vi "translateDigitalInputs.vi"(0 "Controller in":refnum<class "_Controller.lvclass">, 2 "di_value (in)":u32, 5 "error in (no error)":errorcluster) -> (14 "Controller out":refnum<class "_Controller.lvclass">, 16 "dig_in_value (out)":u32, 17 "dig_in_items (out)":T1[](array[typedef]), 19 "error out":errorcluster)   [LabVIEW 2020, in "classes.lvlib" / "_Controller.lvclass"]
uses:
  _Controller.lvclass
  digital_input_item.ctl
  digital_input.ctl
  common.lvlib
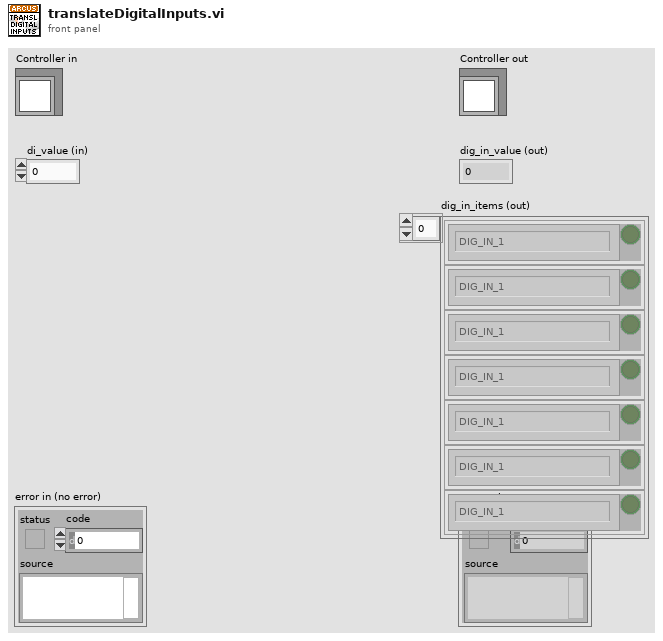
[diagram p1: front panel]
types:
  T1 = typedef "common.lvlib/digital_input_item.ctl" = cluster{"item":T2, "status":bool}
  T2 = typedef "common.lvlib/digital_input.ctl" = enum16{"DIG_IN_1", "DIG_IN_2", "DIG_IN_3", "DIG_IN_4", "DIG_IN_5", "DIG_IN_6", "DIG_IN_7", "DIG_IN_8", "NEG_LIMIT", "HOME", "POS_LIMIT"}
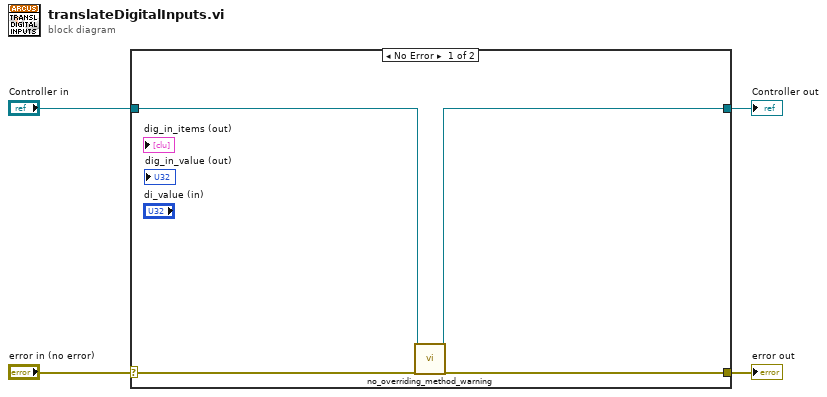
[diagram p0: block diagram]
diagram:
  n1 = case shown="No Error" "error in (no error)" {
    selector: "error in (no error)" -> [w8 w10]
    tunnel: [w7 w10] -> w3
    tunnel: [w5 w9] -> w1
    tunnel: "Controller in" -> [w6 w9]
    frame No Error {
      n2 = call "no_overriding_method_warning.vi"("Controller (in)"=w6, "error in (no error)"=w8) -> ("Controller (out)"=w5:refnum<class "_Controller.lvclass">, "error out"=w7:errorcluster)  [unwired: 15 in, 1 out]
    }
    frame Error {
    }
  }
  "error out" <- w3
  "Controller out" <- w1
